vi "LVFunction_Imop_SlopesCompute_ModalWavefront.vi"(0 "ModalCoef.lvclass":refnum<class "ModalCoef.lvclass">, 1 "ComputePhaseSet":refnum<class "ComputePhaseSet.lvclass">, 2 "HasoSlopes":refnum<class "HasoSlopes.lvclass">, 7 "Phase":refnum<class "Phase.lvclass">, 11 "error constant":errorcluster) -> (4 "ModalCoef.lvclass (dup)":refnum<class "ModalCoef.lvclass">, 8 "Phase (dup)":refnum<class "Phase.lvclass">, 15 "error out":errorcluster)   [LabVIEW 2020]
doc: "Compute phase from slopes via modal coefficients in a given basis of\npolynomials provided by ComputePhaseSet.\n\n--------------------------------------------------------------------------------\n\nHasoDataIn\n HasoData object.\n\nHasoDataOut\n HasoData object.\n\nComputePhaseSet\n cComputePhaseSet object.\n\nphase\n cPhase object.\n\nErrorIn\n Error\nErrorOut\n Error"
uses:
  ComputePhaseSet.lvclass
  Phase.lvclass
  ModalCoef.lvclass
  HasoSlopes.lvclass
  LVClass_ModalCoef Read ModalCoef.vi
  LVClasse_Phase Read SurfaceFloatWithPupil.vi
  LVClass_ComputePhaseSet Read ComputePhaseSet.vi
  LVClass_HasoSlopes Read HasoSlopes _ property.vi
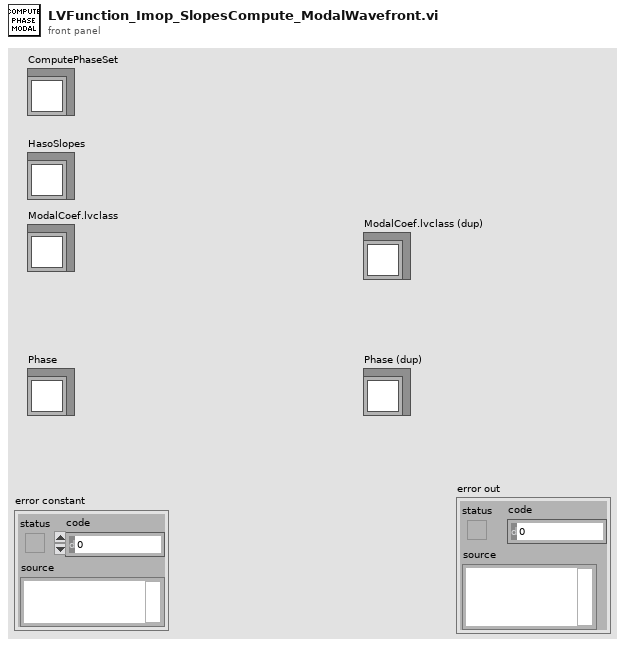
[diagram p1: front panel]
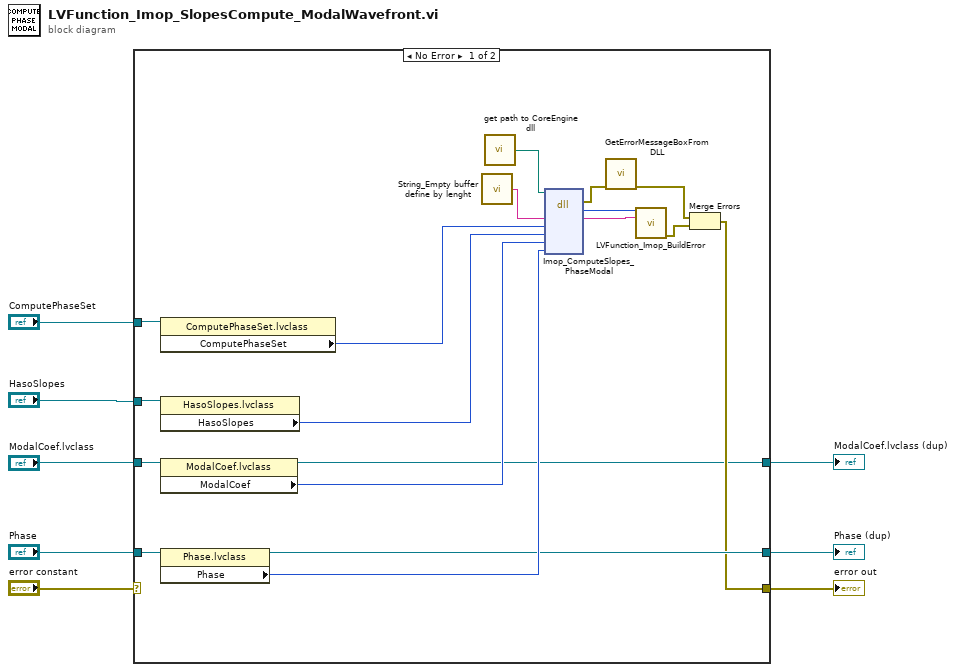
[diagram p0: block diagram]
diagram:
  n1 = case shown="No Error" "error constant" {
    selector: "error constant" -> [_ w29]
    tunnel: "HasoSlopes" -> [w21 _]
    tunnel: "ComputePhaseSet" -> [w20 _]
    tunnel: [w12 w29] -> w7
    tunnel: "Phase" -> [w19 w28]
    tunnel: [w15 w28] -> w4
    tunnel: "ModalCoef.lvclass" -> [w10 w27]
    tunnel: [w9 w27] -> w2
    frame No Error {
      n2 = property class="ComputePhaseSet.lvclass"(reference=w20) -> ("ComputePhaseSet"=w17:i32)  [unwired: 1 in, 2 out]
      n3 = property class="HasoSlopes.lvclass"(reference=w21) -> ("HasoSlopes"=w18:i32)  [unwired: 1 in, 2 out]
      n4 = property class="ModalCoef.lvclass"(reference=w10) -> (reference out=w9:refnum<class "ModalCoef.lvclass">, "ModalCoef"=w11:u32)  [unwired: 1 in, 1 out]
      n5 = property class="Phase.lvclass"(reference=w19) -> (reference out=w15:refnum<class "Phase.lvclass">, "Phase"=w16:i32)  [unwired: 1 in, 1 out]
      n6 = call "String_Empty buffer define by lenght.vi"() -> ("Empty buffer"=w24:string)  [unwired: 1 in]
      n7 = call "get path to CoreEngine dll.vi"() -> ("path to c_interface_vc100.dll"=w23:path)  [unwired: 12 in, 3 out]
      n8 = dll-call lib="D:/FLE/0.Code/CoreEngine4_Suite/LV2011_interface/DLLs/c_interface_vc100.dll" fn="Imop_ComputeSlopes_PhaseModal"(path in=w23, "message"=w24, "ComputePhaseSet"=w17, "HasoSlopes"=w18, "ModalCoeffs"=w11, "Phase"=w16) -> (error out=w22:errorcluster, "return type"=w26:i32, "message"=w25:string)  [unwired: 6 in, 1 out]
      n9 = call "GetErrorMessageBoxFromDLL.vi"("error IN"=w22) -> ("error OUT"=w14:errorcluster)  [unwired: 10 in]
      n10 = call "LVFunction_Imop_BuildError.vi"("code"=w26, "String to Prepend to source (\"\")"=w25) -> ("error out"=w13:errorcluster)  [unwired: 13 in]
      n11 = Merge Errors(w14, w13) -> (w12:errorcluster)
    }
    frame Error {
    }
  }
  "error out" <- w7
  "Phase (dup)" <- w4
  "ModalCoef.lvclass (dup)" <- w2
